vi "Send Shortcut Menu Selection.vi"(0 "Message Enqueuer in":refnum<class "Message Enqueuer.lvclass">, 1 "App Item?":bool, 3 "EventFilter Reference":T1, 5 "CtlRef":refnum<vi>, 7 "Time":u32, 9 "Item Tag":string, 11 "Item Path":string, 12 "Coords":T2, 13 "SubObj":refnum<vi>) -> (4 "Filtered EventDataMessage":refnum<class "ShortcutMenuSelectionMsg.lvclass">, 15 "error out":errorcluster)   [LabVIEW 2015, in "ActorEvents.lvlib" / "ShortcutMenuSelectionMsg.lvclass"]
doc: "<License>\nCopyright © 2017 Composed Systems, LLC | All rights reserved\nwww.composed.io\n\nAuthor: Ethan Stern <ethan.stern@composed.io>\n\nThis software is provided \"AS IS\" WITHOUT WARRANTIES, either express or implied, AND IS FOR EDUCATIONAL PURPOSES ONLY.\n</License>"
uses:
  ShortcutMenuSelectionMsg.lvclass
  <vilib>/ActorFramework/Message Enqueuer/Message Enqueuer.lvclass
  <vilib>/Utility/miscctls.llb/LVPoint32TypeDef.ctl
  IEventFilter/EventFilter Reference.ctl
  IEventFilter/IEventFilter.lvclass
  ShortcutMenuSelectionMsg.lvclass/ShortcutMenuSelectionMsg.ctl
  EventDataMessage/EventDataMessage.lvclass/EventDataMessage.ctl
  <vilib>/ActorFramework/Message Enqueuer/Message Enqueuer.lvclass/Message Enqueuer.ctl
  <vilib>/ActorFramework/Message Enqueuer/Enqueue.vi
  <vilib>/Utility/error.llb/Clear Errors.vi
  <vilib>/ActorFramework/Message Priority Queue/Priority Enqueue.vi
  EventDataMessage/EventDataMessage.lvclass
panel:
  in  "error in (no error)":errorcluster
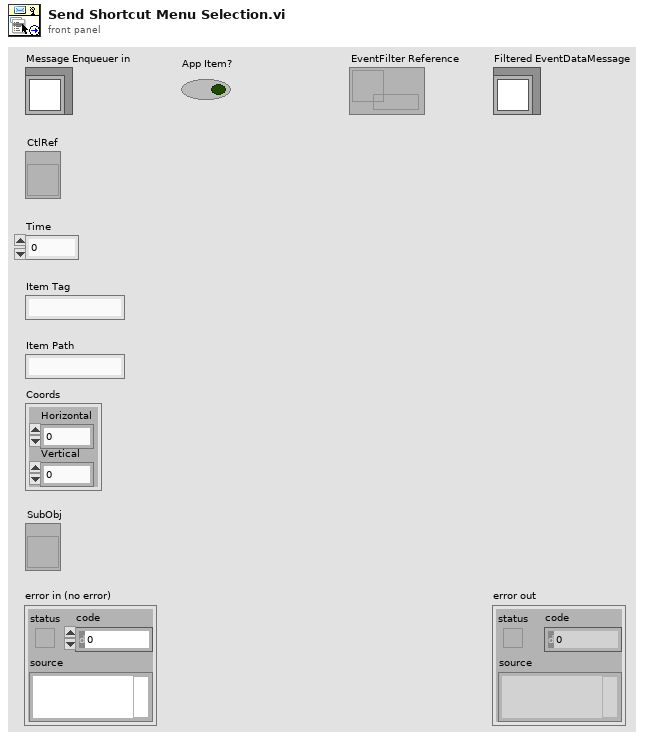
[diagram p1: front panel]
types:
  T1 = typedef "ActorEvents.lvlib/IEventFilter.lvclass/EventFilter Reference.ctl" = refnum<data-value>
  T2 = typedef "LVPoint32TypeDef.ctl" = cluster{"Horizontal":i32, "Vertical":i32}
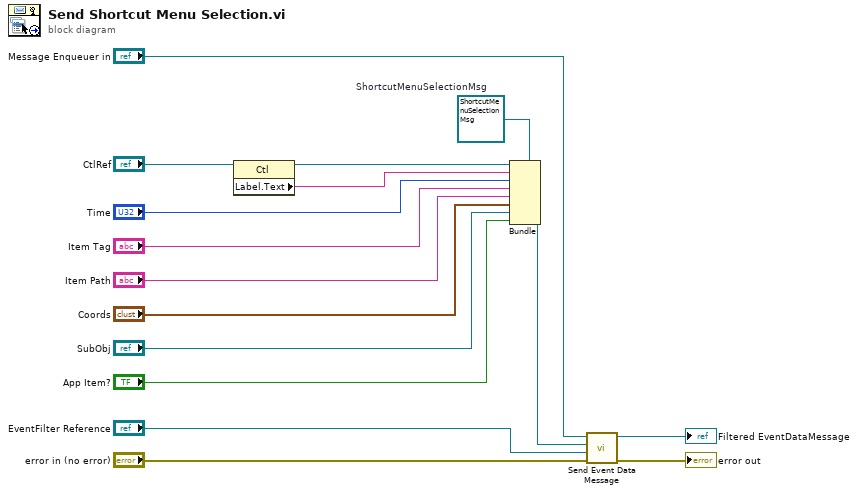
[diagram p0: block diagram]
diagram:
  w16 = refnum<class "ShortcutMenuSelectionMsg.lvclass"> refnum  # ShortcutMenuSelectionMsg
  n1 = property class="Ctl"(reference="CtlRef") -> (reference out=w10:refnum<vi>, "Label.Text"=w4:string)  [unwired: 1 in, 1 out]
  n2 = Bundle(cluster=w16, w10, w4, "Time", "Item Tag", "Item Path", "Coords", "SubObj", "App Item?") -> (w13:refnum<class "ShortcutMenuSelectionMsg.lvclass">)
  n3 = call "Send Event Data Message.vi"("error in (no error)"="error in (no error)", "EventFilter Reference"="EventFilter Reference", "EventDataMessage"=w13, "Message Enqueuer in"="Message Enqueuer in") -> ("error out"=→"error out":errorcluster, "Filtered EventDataMessage"=→"Filtered EventDataMessage":refnum<class "ShortcutMenuSelectionMsg.lvclass">)  [unwired: 6 in]
